vi "CoordSystem_Convert_Transform3d.vi"(9 "CoordSys To":T1={"Rotation"={"Q_quaternion"={"R"=1.0, "V"=[0.0, 0.0, 0.0]}}}, 10 "CoordSys From":T1={"Rotation"={"Q_quaternion"={"R"=1.0, "V"=[0.0, 0.0, 0.0]}}}, 11 "in Transform3d":T4={"TRANSLATION3D"={"X"=0.0, "Y"=0.0, "Z"=0.0}, "ROTATION3D"={"Q_quaternion"={"R"=1.0, "V"=[0.0, 0.0, 0.0]}}, "XF"=FALSE} {"TRANSLATION3D"."Z" format="%14.3f"; "TRANSLATION3D"."Y" format="%14.3f"; "TRANSLATION3D"."X" format="%14.3f"}) -> (3 "out Converted Transform3d":T4={"TRANSLATION3D"={"X"=0.0, "Y"=0.0, "Z"=0.0}, "ROTATION3D"={"Q_quaternion"={"R"=1.0, "V"=[0.0, 0.0, 0.0]}}, "XF"=FALSE} {"TRANSLATION3D"."Z" format="%14.3f"; "TRANSLATION3D"."Y" format="%14.3f"; "TRANSLATION3D"."X" format="%14.3f"})   [LabVIEW 2019, in "Trajectory_Library.lvlib"]
doc: "Converts the given transform3d from one coordinate system to another.\n\nInputs:\n - in transform3d -- The transform3d to convert.\n - Coord Sys from -- The coordinate system the pose starts in.\n - Coord Sys to -- The coordinate system to which to convert.\n\nReturns:\n - Converted transform3d -- The given transform3d in the desired coordinate system."
uses:
  TypeDef/TRANSLATION3D.ctl
  TypeDef/ROTATION3D.ctl
  TypeDef/QUATERNION.ctl
  TypeDef/COORDINATE_SYSTEM.ctl
  Rotation3d_UnaryMinus.vi
  Rotation3d_RotateBy.vi
  Transform3d_Create_Pose3dPose3d.vi
  Transform3d_GetRotation3d.vi
  Transform3d_GetTranslation3d.vi
  Rotation3d_Create_Quaternion.vi
  Quaternion_Inverse.vi
  Rotation3d_GetQuaterion.vi
  Quaternion_Times.vi
  Translation3d_Minus.vi
  Translation3d_RotateBy.vi
  Pose3d_getTranslation3d.vi
  Pose3d_getRotation3d.vi
  Quaternion_Normalize.vi
  Translation3d_Create.vi
  Quaternion_New.vi
  Quaternion_Get_All.vi
  Quaternion_New_Default.vi
  Trajectory_Library.lvlib
  TypeDef/TRANSFORM3D.ctl
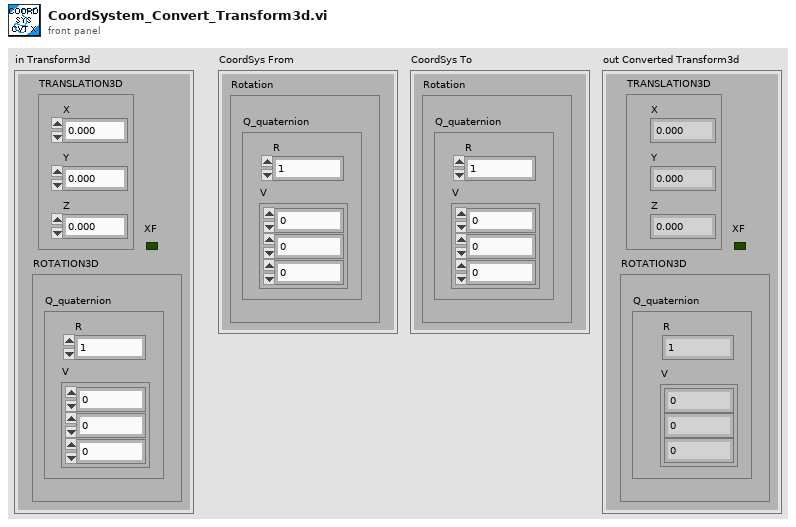
[diagram p1: front panel]
types:
  T1 = typedef "Trajectory_Library.lvlib/COORDINATE_SYSTEM.ctl" = cluster{"Rotation":T2}
  T2 = typedef "Trajectory_Library.lvlib/ROTATION3D.ctl" = cluster{"Q_quaternion":T3}
  T3 = typedef "Trajectory_Library.lvlib/QUATERNION.ctl" = cluster{"R":dbl, "V":dbl[]}
  T4 = typedef "Trajectory_Library.lvlib/TRANSFORM3D.ctl" = cluster{"TRANSLATION3D":T5, "ROTATION3D":T2, "XF":bool}
  T5 = typedef "Trajectory_Library.lvlib/TRANSLATION3D.ctl" = cluster{"X":dbl, "Y":dbl, "Z":dbl}
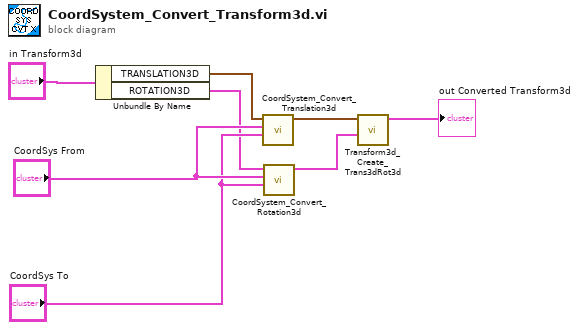
[diagram p0: block diagram]
diagram:
  n1 = Unbundle By Name("in Transform3d") -> ("TRANSLATION3D"=w5:T5, "ROTATION3D"=w4:T2)
  n2 = call "CoordSystem_Convert_Translation3d.vi"("CoordSys To"="CoordSys To", "CoordSys From"="CoordSys From", "in Translation3d"=w5) -> ("out Converted Translation3d"=w3:T5)  [unwired: 8 in]
  n3 = call "CoordSystem_Convert_Rotation3d.vi"("CoordSys To"="CoordSys To", "CoordSys From"="CoordSys From", "in Rotation3d"=w4) -> ("out Converted Rotation3d"=w2:T2)  [unwired: 8 in]
  n4 = call "Transform3d_Create_Trans3dRot3d.vi"("Rotation3d"=w2, "Translation3d"=w3) -> ("Transform3d"=→"out Converted Transform3d":T4)  [unwired: 9 in]
